vi "EloMec Tester.vi"() -> ()   [LabVIEW 2022 SP3]
uses:
  Communication_class/Paths/Convert AI Robot to Robot Command Folder/grSim/grSim Robot Command.ctl
  <vilib>/Instr/_visa.llb/VISA Configure Serial Port (Instr).vi
  Communication_class/Communication.lvclass
panel:
  in  "Wheel":sgl[](array[numeric])
  in  "Feedback ID":u32
  out "Waveform Chart":T1(graph)
  in  "IDs":u32[](array[numeric])=[0, 1, 2, 3, 4, 5, 6]
  out "Numeric 2":u32
  out "String":string
  out "return count":u32
  in  "stop":bool
  out "string":string
  out "error out":errorcluster
  in  "termination char\n(0xA = '\\n' = LF)":u8=10 format="%.0x"
  in  "VISA resource name":refnum<visa-resource-name>
  in  "Serial Settings":T2={"baud rate"=9600, "data bits"=8, "parity"=enum."None", "stop bits"=10, "flow control"=0} {"flow control" items=["None"=0, "XON/XOFF"=1, "RTS/CTS"=2, "DTR/DSR"=4]; "stop bits" items=["1"=10, "1.5"=15, "2.0"=20]; "data bits" min=5 max=8 step=1; "baud rate" items=["75"=75, "110"=110, "134"=134, "150"=150, "300"=300, "600"=600, "1200"=1200, "1800"=1800, "2400"=2400, "4800"=4800, "7200"=7200, "9600"=9600, "14400"=14400, "19200"=19200, "28800"=28800, "38400"=38400, "56000"=56000, "57600"=57600, "115200"=115200, "128000"=128000, "230400"=230400]}
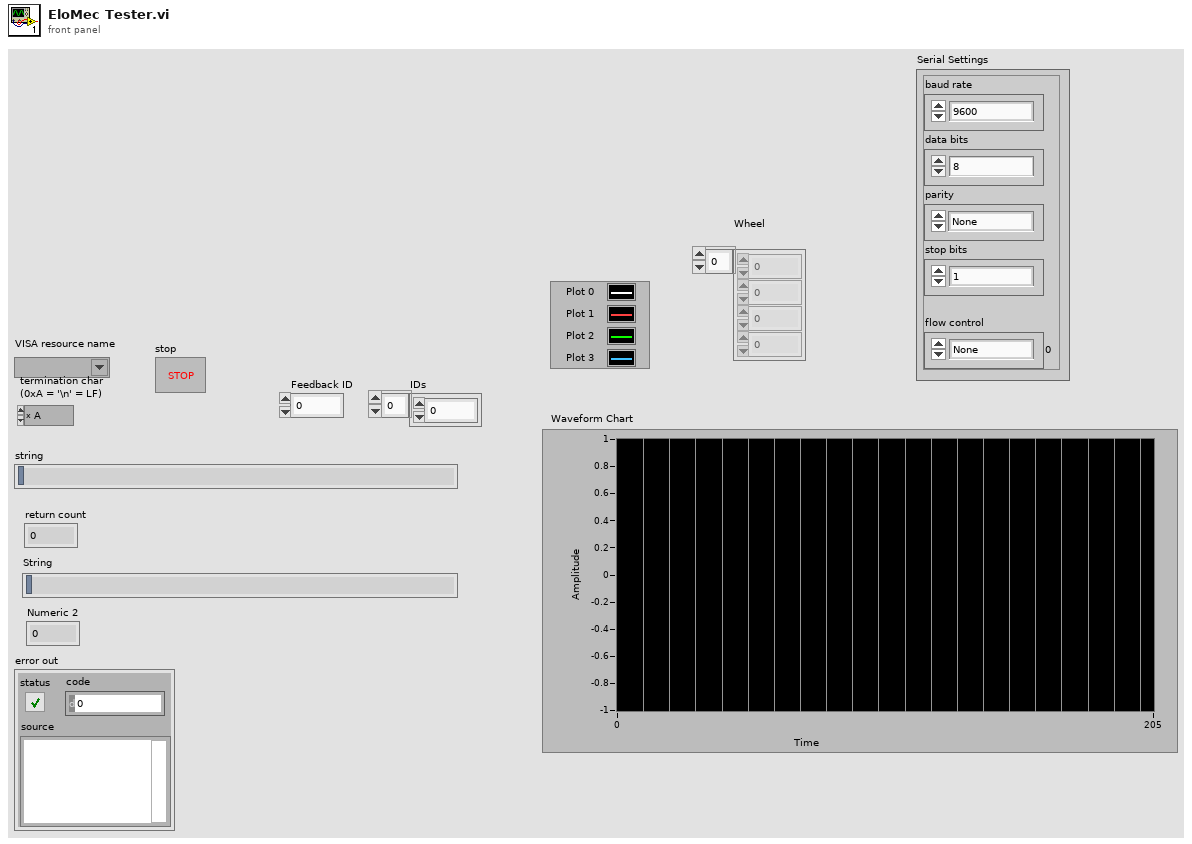
[diagram p1: front panel]
types:
  T1 = cluster{"[0]":sgl, "[1]":sgl, "[2]":sgl, "[3]":sgl, "[4]":sgl, "[5]":sgl, "[6]":sgl, "[7]":sgl, "[8]":sgl}
  T2 = cluster{"baud rate":u32, "data bits":u16, "parity":enum16{"None", "Odd", "Even", "Mark", "Space"}, "stop bits":u16, "flow control":u16}
  T3 = typedef "grSim Robot Command.ctl" = cluster{"id":u32, "kickspeedx":sgl, "kickspeedz":sgl, "veltangent":sgl, "velnormal":sgl, "velangular":sgl, "spinner":bool, "wheelspeed":bool, "wheel1":sgl, "wheel2":sgl, "wheel3":sgl, "wheel4":sgl, "kickangle":sgl, "spinner_rpm":sgl}
  T4 = typedef "feedbackData.ctl" = cluster{"id":u32, "status":u32, "battery":sgl, "encoder1":sgl, "encoder2":sgl, "encoder3":sgl, "encoder4":sgl}
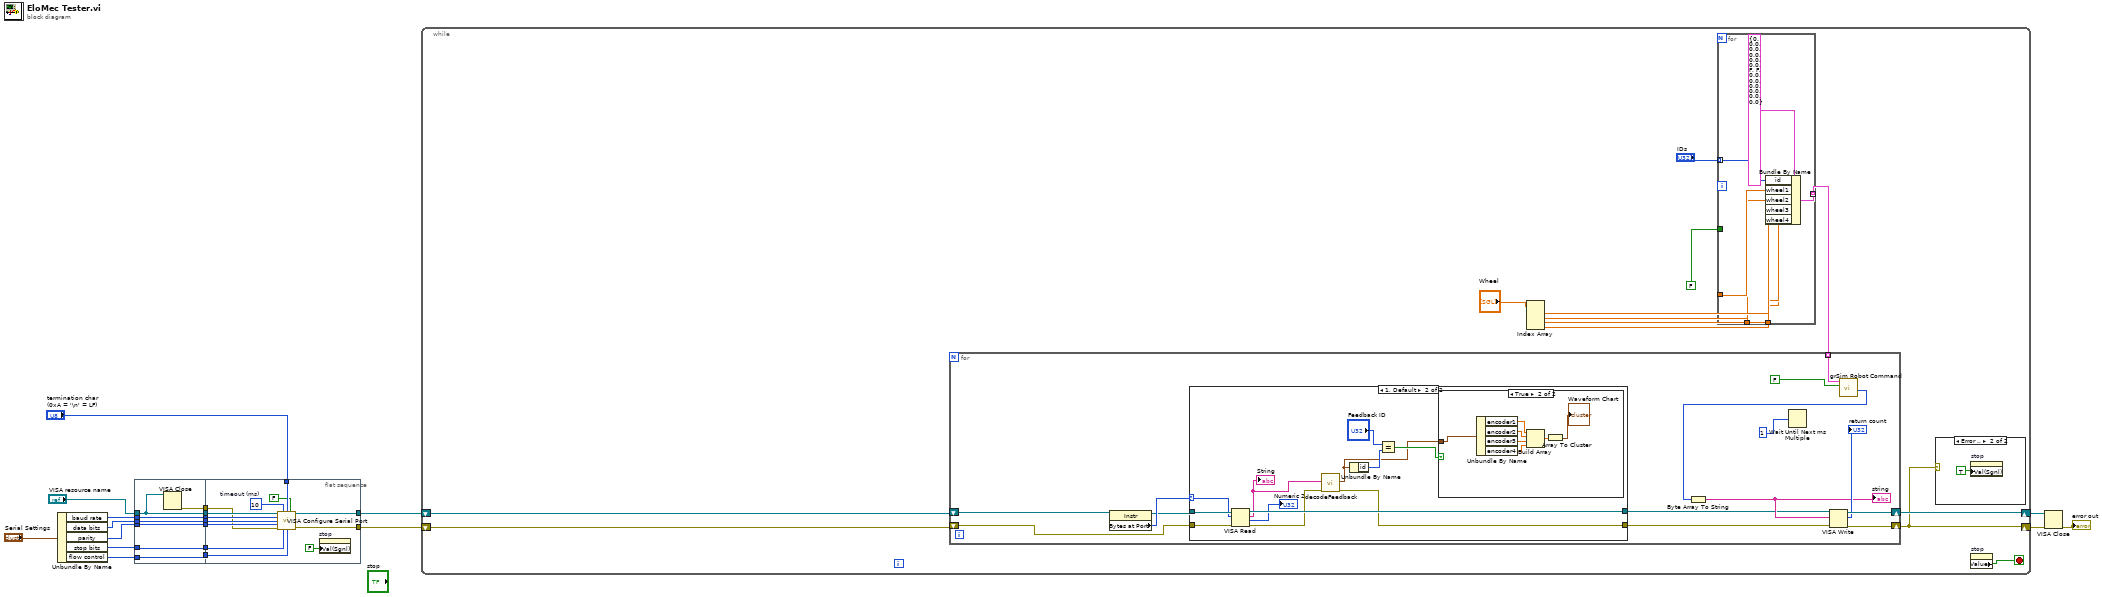
[diagram p0: block diagram]
diagram:
  n1 = Unbundle By Name("Serial Settings") -> ("baud rate"=w19:u32, "data bits"=w18:u16, "parity"=w17:enum16{"None", "Odd", "Even", "Mark", "Space"}, "stop bits"=w16:u16, "flow control"=w15:u16)
  n2 = flat-sequence {
    tunnel: "VISA resource name" -> [w22]
    tunnel: w15 -> [w23]
    tunnel: w16 -> [w24]
    tunnel: w17 -> [w25]
    tunnel: w18 -> [w26]
    tunnel: w19 -> [w27]
    tunnel: [w27] -> w7
    tunnel: [w26] -> w6
    tunnel: [w25] -> w5
    tunnel: [w24] -> w4
    tunnel: [w23] -> w3
    tunnel: [w22] -> w2
    tunnel: [w21] -> w1
    tunnel: "termination char\n(0xA = '\\n' = LF)" -> [w34]
    tunnel: [w32] -> w12
    tunnel: [w31] -> w10
    tunnel: w7 -> [w40]
    tunnel: w6 -> [w39]
    tunnel: w5 -> [w38]
    tunnel: w4 -> [w37]
    tunnel: w3 -> [w36]
    tunnel: w2 -> [w35]
    tunnel: w1 -> [w29]
    frame #0 {
      n3 = VISA Close(VISA resource name=w22) -> (error out=w21:errorcluster)  [unwired: 1 in]
    }
    frame #1 {
      w30 = u32 10  # timeout (ms)
      n4 = call-poly "VISA Configure Serial Port"("VISA resource name"=w35, "timeout (10sec)"=w30, "termination char\n(0xA = '\\n' = LF)"=w34, "Enable Termination\nChar (T)"=FALSE ("Enable Termination\nChar (T)"), "baud rate (9600)"=w40, "data bits (8)"=w39, "parity (0:none)"=w38, "error in (no error)"=w29, "stop bits (10: 1 bit)"=w37, "flow control (0:none)"=w36) -> ("VISA resource name out"=w32:refnum<visa-resource-name>, "error out"=w31:errorcluster)  [unwired: 4 in]
      n5 = property on="stop" class="Bool (strict)"("Val(Sgnl)"=FALSE ("Value (Signaling)")) -> ()  [unwired: 2 in, 2 out]
    }
  }
  n6 = while {
    shift-right: [w53] -> w11
    shift-left: w12 -> [w47]
    shift-right: [w48] -> w9
    shift-left: w10 -> [w46]
    stop <- w49 stop-if-true
    n7 = Index Array(array="Wheel") -> (element #1=w44:sgl, element #2=w43:sgl, element #3=w42:sgl, element #4=w41:sgl)  [unwired: 4 in]
    n8 = for {
      tunnel: FALSE -> [_]
      tunnel: [w96] -> w50 mode=indexing
      tunnel: "IDs" -> [w94] mode=indexing
      tunnel: [w93] -> _
      tunnel: w44 -> [w93]
      tunnel: w43 -> [w92]
      tunnel: w42 -> [w91]
      tunnel: w41 -> [w90]
      n9 = Bundle By Name(cluster=T3 {"id"=0, "kickspeedx"=0.0, "kickspeedz"=0.0, "veltangent"=0.0, "velnormal"=0.0, "velangular"=0.0, "spinner"=FALSE, "wheelspeed"=FALSE, "wheel1"=0.0, "wheel2"=0.0, "wheel3"=0.0, "wheel4"=0.0, "kickangle"=0.0, "spinner_rpm"=0.0} ("Robots"), "id"=w94, "wheel1"=w93, "wheel2"=w92, "wheel3"=w91, "wheel4"=w90) -> (w96:T3)
    }
    n10 = for {
      shift-right: [w66] -> w48
      shift-left: w46 -> [w58]
      shift-right: [w68] -> w53
      shift-left: w47 -> [w59]
      tunnel: w50 -> [w63] mode=indexing
      n11 = property class="Instr"(reference=w59) -> (reference out=w57:refnum<visa-resource-name>, "Bytes at Port"=w62:u32)  [unwired: 1 in, 1 out]
      n12 = case shown="1, Default" w62 {
        selector: w62 -> [_ w72]
        tunnel: w58 -> [w69 w82]
        tunnel: [w69 w78] -> w61
        tunnel: w57 -> [w70 w73]
        tunnel: [w70 w81] -> w60
        frame 0 {
        }
        frame 1, Default {
          n13 = VISA Read(VISA resource name=w73, byte count=w72, error in (no error)=w82) -> (VISA resource name out=w81:refnum<visa-resource-name>, read buffer=w80:string, return count=→"Numeric 2":u32, error out=w79:errorcluster)
          "String" <- w80
          n14 = call "decodeFeedback.vi"("error in (no error)"=w79, "String"=w80) -> ("error out"=w78:errorcluster, "FeedbackData"=w74:T4)  [unwired: 7 in, 1 out]
          n15 = Unbundle By Name(w74) -> ("id"=w76:u32)
          n16 = Equal?(x="Feedback ID", y=w76) -> (x = y?=w75:bool)
          n17 = case shown="True" w75 {
            tunnel: w74 -> [_ w84]
            frame False {
            }
            frame True {
              n18 = Unbundle By Name(w84) -> ("encoder1"=w83:sgl, "encoder2"=w89:sgl, "encoder3"=w88:sgl, "encoder4"=w87:sgl)
              n19 = Build Array(w83, w89, w88, w87) -> (w86:sgl[])
              n20 = Array To Cluster(array=w86) -> (cluster=→"Waveform Chart":T1)
            }
          }
        }
      }
      n21 = Wait Until Next ms Multiple(millisecond multiple=u32 1 ("milliseconds to wait")) -> ()  [unwired: 1 out]
      n22 = call "grSim Robot Command.vi"("FIRASim?"=FALSE, "Robots"=w63) -> ("Array"=w64:u8[])  [unwired: 9 in]
      n23 = Byte Array To String(unsigned byte array=w64) -> (string=w65:string)
      "string" <- w65
      n24 = VISA Write(VISA resource name=w60, write buffer=w65, error in (no error)=w61) -> (VISA resource name out=w68:refnum<visa-resource-name>, return count=→"return count":u32, error out=w66:errorcluster)
    }
    n25 = case shown="Error .." w48 {
      frame No Error {
      }
      frame Error {
        n26 = property on="stop" class="Bool (strict)"("Val(Sgnl)"=TRUE ("Value (Signaling)")) -> ()  [unwired: 2 in, 2 out]
      }
    }
    n27 = property on="stop" class="Bool (strict)"() -> ("Value"=w49:bool)  [unwired: 2 in, 2 out]
  }
  n28 = VISA Close(VISA resource name=w11, error in (no error)=w9) -> (error out=→"error out":errorcluster)
